vi "Test-Shoulder.vi"() -> ()   [LabVIEW 2023]
doc: "This VI implements the framework and scheduler for your robotics program. It should not be necessary to modify the framework. You are expected to add your code to the VIs called from Robot Main - the ones located in the Team Code folder within the project."
uses:
  <vilib>/Rock Robotics/WPI/DriverStation/WPI_DriverStationRobotMode2.ctl
  <vilib>/Rock Robotics/WPI/Simulation/Protocol/Devices/DriverStation/DS Update Ops.ctl
  <vilib>/Rock Robotics/WPI/ThirdParty/JAS_Junk/TrajLib/VI/DigSeqLogic_Edge_On.vi
  Robot Global Data.vi
  Shoulder/ShoulderCmdCalcSpeakerShootALWAYS.vi
  Shoulder/ShoulderCmdUpIncALWAYS.vi
  Shoulder/ShoulderCmdDownDecALWAYS.vi
  Shoulder/ShoulderCmdRestALWAYS.vi
  Shoulder/ShoulderCmdSpeakerShootALWAYS.vi
  Shoulder/ShoulderCmdStopALWAYS.vi
  Shoulder/ShoulderCmdAmpDeliverALWAYS.vi
panel:
  in  "CmdInc":bool
  in  "CmdDec":bool
  in  "CmdStop":bool
  out "Low Limit Switch":bool
  out "PosDeg":dbl format="%9.1f"
  in  "CmdRest":bool
  in  "CmdAmp":bool
  in  "CmdSpeaker":bool
  in  "CmdCalcSpeaker":bool
  out "Robot Mode":T1
  out "MotorOutDmd":dbl format="%9.2f"
  in  "error in (no error)":errorcluster
  in  "Finish":bool
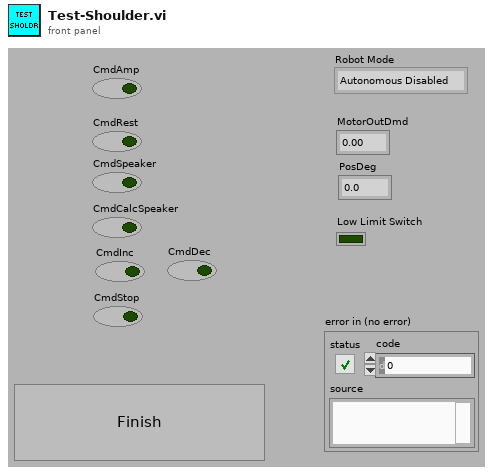
[diagram p1: front panel]
types:
  T1 = typedef "WPI_DriverStationRobotMode2.ctl" = enum16{"Autonomous Disabled", "Autonomous Enabled", "Teleop Disabled", "Teleop Enabled", "Disconnected", "Finish", "Test Disabled", "Test Enabled", "Emergency Stopped"}
  T2 = typedef "WPI_DriverStationMatch Info.ctl" = cluster{"Autonomous Elapsed Seconds":dbl, "TeleOp Elapsed Seconds":dbl, "Disabled Elapsed Seconds":dbl, "Visited Autonomous":bool, "Visited TeleOp":bool, "Visited Disabled":bool, "Autonomous Settings":cluster{"Autonomous Style":enum16{"Iterative", "Independent"}, "VI Refnum":refnum<vi>}}
  T3 = typedef "WPI_DriverStationDerivedRobotMode.ctl" = enum16{"Init", "Execute", "Stop"}
  T4 = typedef "DS Update Ops.ctl" = enum16{"set enabled", "set autonomous", "set test", "set estop", "set fms", "set ds", "set control word", "set match_time", "set station", "set game data", "JSON update", "set name", "get", "transmit initial", "reset"}
  T5 = typedef "NetComm_ControlWord.ctl" = cluster{"Enabled":bool, "Autonomous":bool, "Test":bool, "E-Stop":bool, "FMS Attached":bool, "DS Attached":bool}
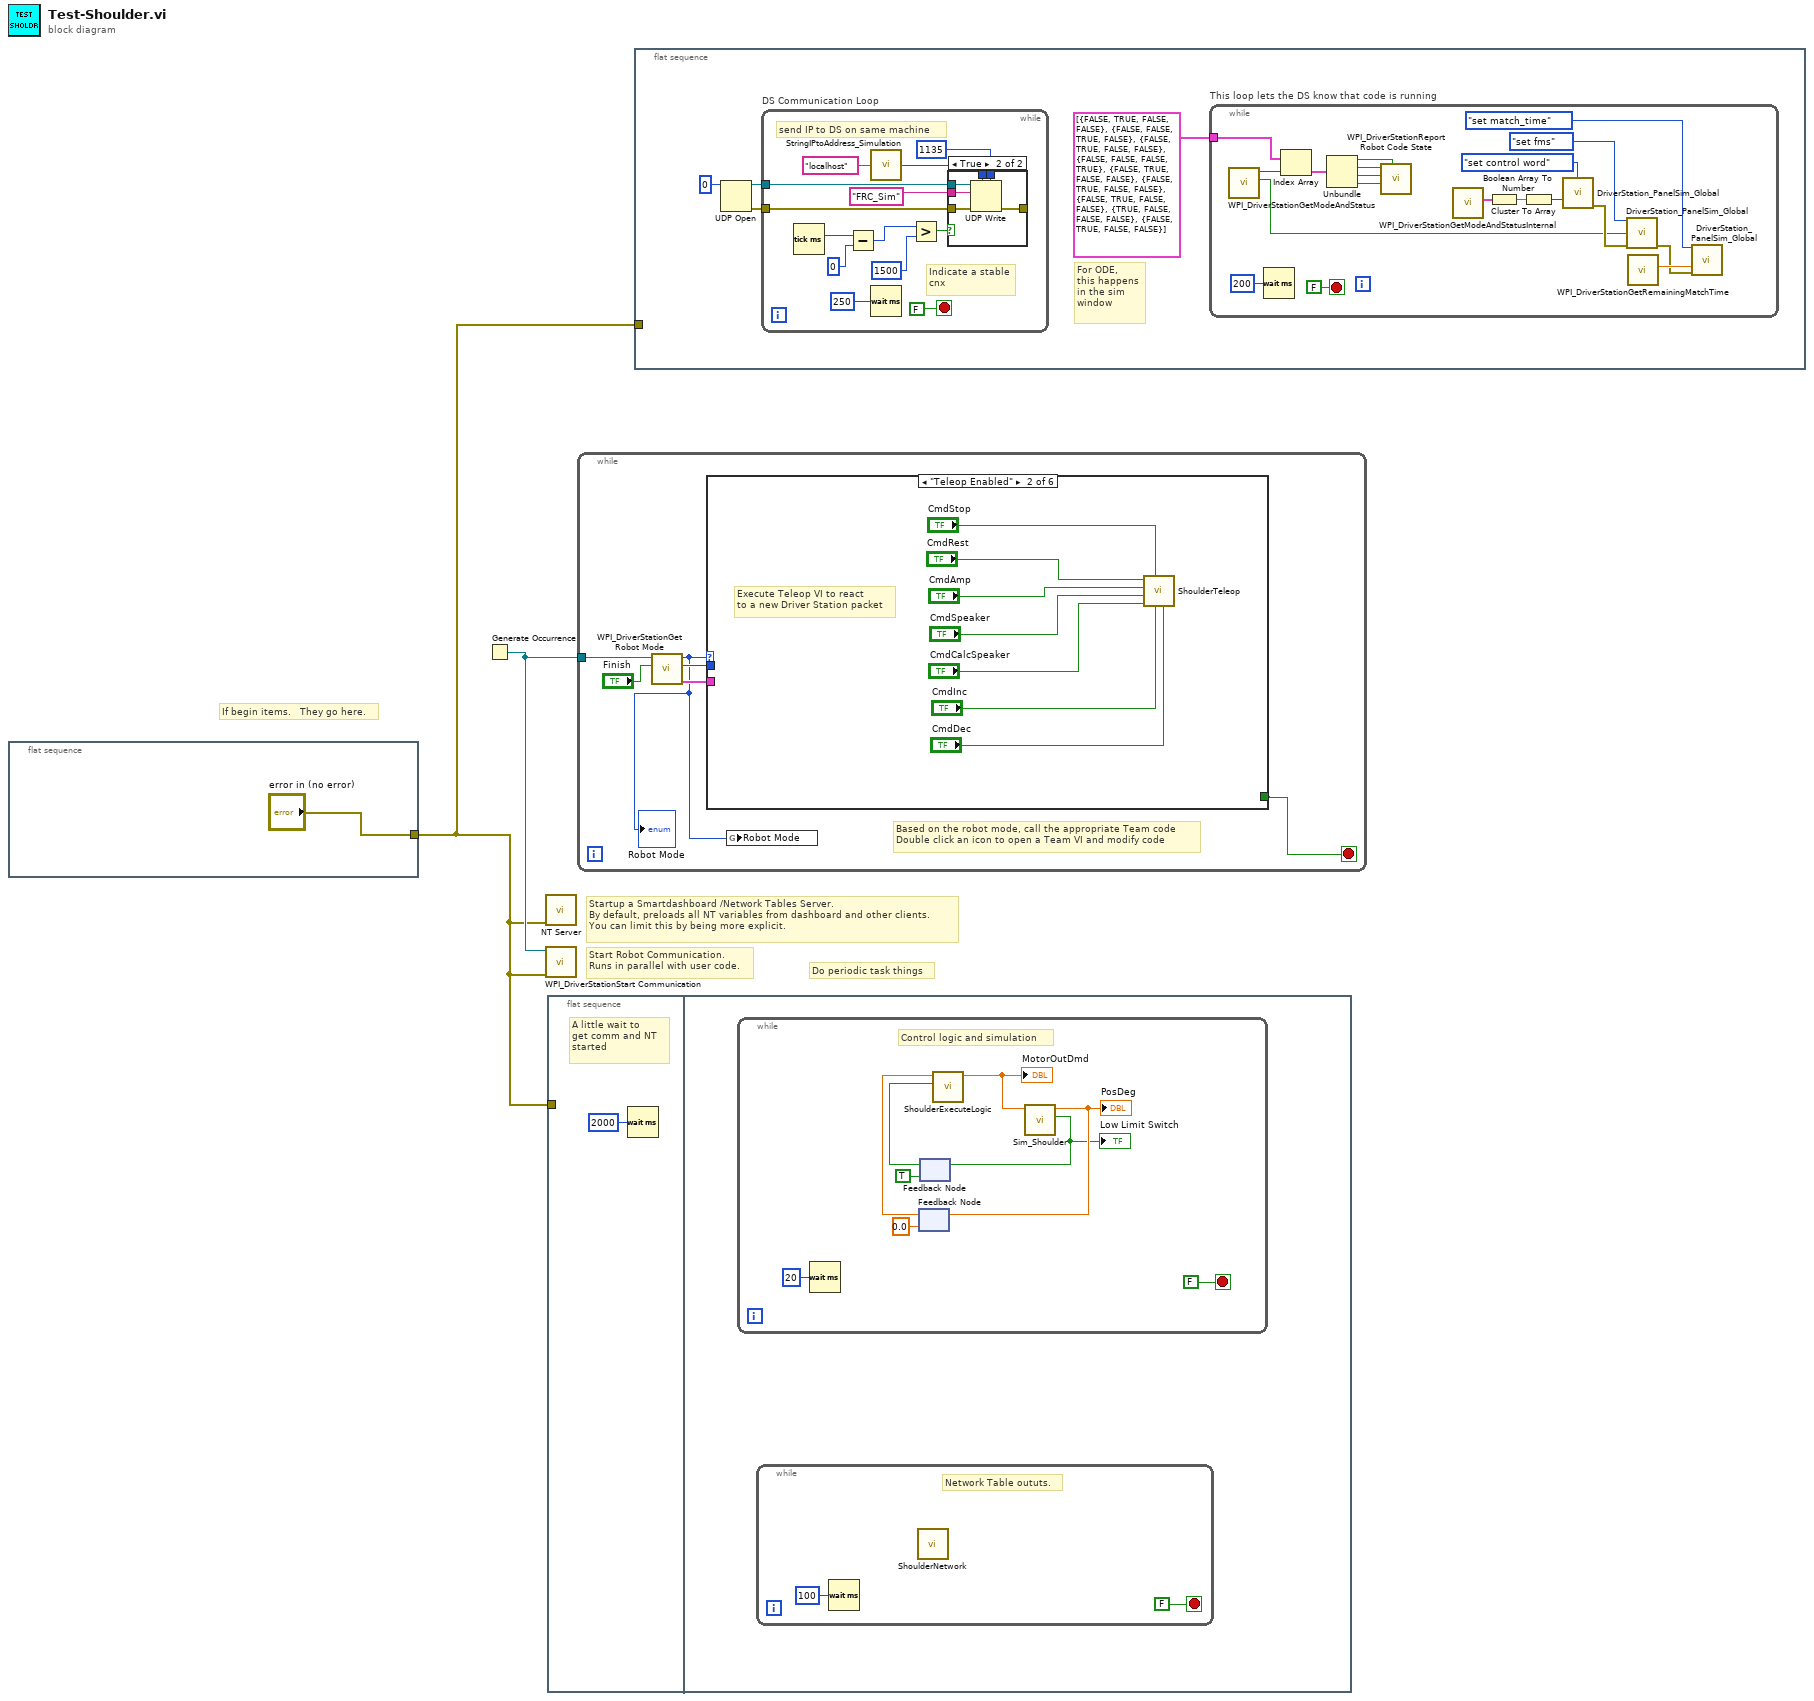
[diagram p0: block diagram]
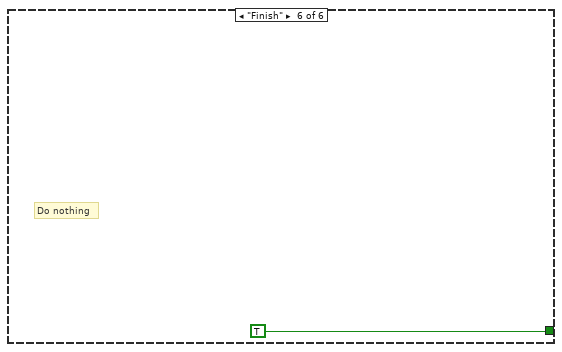
[diagram p6: hidden frame]
diagram:
  # "If begin items.   They go here."
  # "Do periodic task things"
  # "Startup a Smartdashboard /Network Tables Server.\nBy default, preloads all NT variables from dashboard and other clients.\nYou can limit this by being more explicit."
  # "Start Robot Communication.\nRuns in parallel with user code."
  n1 = flat-sequence {
    tunnel: ["error in (no error)"] -> w1
    frame #0 {
    }
  }
  n2 = Generate Occurrence() -> (w2:refnum<k4>)
  n3 = call <vilib>:"NT Server.vi"("error in (no error)"=w1) -> ()  [unwired: 10 in, 1 out]
  n4 = call <vilib>:"WPI_DriverStationStart Communication.vi"("error in (no error)"=w1, "occurrence"=w2) -> ()  [unwired: 1 in, 9 out]
  n5 = flat-sequence {
    tunnel: w1 -> [_]
    frame #0 {
      # "A little wait to\nget comm and NT\nstarted"
      n6 = Wait (ms)(milliseconds to wait=u32 2000) -> ()  [unwired: 1 out]
    }
    frame #1 {
      n7 = while {
        stop <- FALSE stop-if-true
        # "Control logic and simulation"
        n8 = Wait (ms)(milliseconds to wait=u32 20) -> ()  [unwired: 1 out]
        n9 = feedback #1(0.0 ("ArmPosDeg")) -> (w11:dbl)
        n10 = feedback #2(TRUE ("Low Limit Switch")) -> (w9:bool)
        n11 = call "ShoulderExecuteLogic.vi"("LowLimitSwitch"=w9, "PositionDeg"=w11) -> ("MotorDemand"=w13:dbl)  [unwired: 8 in, 1 out]
        "MotorOutDmd" <- w13
        n12 = call "Sim_Shoulder.vi"("Motor Dmd"=w13) -> ("Low Limit Switch"=w10:bool, "ArmPosDeg"=w12:dbl)  [unwired: 8 in, 1 out]
        "PosDeg" <- w12
        "Low Limit Switch" <- w10
        n13 = feedback-in #1(w12) -> ()
        n14 = feedback-in #2(w10) -> ()
      }
      n15 = while {
        stop <- FALSE stop-if-true
        # "Network Table oututs."
        n16 = Wait (ms)(milliseconds to wait=u32 100) -> ()  [unwired: 1 out]
        n17 = call "ShoulderNetwork.vi"() -> ()  [unwired: 11 in, 1 out]
      }
    }
  }
  n18 = while {
    tunnel: w2 -> [w21]
    stop <- w16 stop-if-true
    # "Based on the robot mode, call the appropriate Team code\nDouble click an icon to open a Team VI and modify code"
    n19 = call <vilib>:"WPI_DriverStationGet Robot Mode.vi"("Finish"="Finish", "DS Occurrence"=w21) -> ("Match Info out"=w18:T2, "Call Context"=w20:T3, "Robot Mode"=w17:T1)  [unwired: 7 out]
    "Robot Mode" <- w17
    n20 = case shown="\"Teleop Enabled\"" w17 {
      tunnel: w20 -> [_ _ _ _ _ _]
      tunnel: w18 -> [_ _ _ _ _ _]
      tunnel: [_ _ _ _ _ TRUE] -> w16
      frame "Autonomous Enabled" {
        # "Do nothing...."
      }
      frame "Teleop Enabled" {
        # "Execute Teleop VI to react\nto a new Driver Station packet"
        n21 = call "ShoulderTeleop.vi"("CmdDownDec"="CmdDec", "CmdUpInc"="CmdInc", "CmdStop"="CmdStop", "CmdCalcSpeaker"="CmdCalcSpeaker", "CmdSpeaker"="CmdSpeaker", "CmdAmp"="CmdAmp", "CmdRest"="CmdRest") -> ()  [unwired: 5 in]
      }
      frame "Test Disabled", "Test Enabled" {
        # "Do nothing"
      }
      frame "Autonomous Disabled", "Teleop Disabled" {
        # "Do nothing."
      }
      frame "Disconnected", Default {
        # "Driver Station packet didn't arrive.\nPossibly useful for diagnostics"
      }
      frame "Finish" {
        # "Do nothing"
      }
    }
    n22 = global write "Robot Global Data.vi" "Robot Mode"(w17) -> ()
  }
  n23 = flat-sequence {
    tunnel: w1 -> [_]
    frame #0 {
      # "For ODE,\nthis happens\nin the sim\nwindow"
      n24 = UDP Open(11:u16 0 ("port")) -> (port=w33:refnum<k16>, 0:w32:errorcluster)  [unwired: 4 in, 1 out]
      n25 = while "DS Communication Loop" {
        tunnel: w33 -> [w64]
        tunnel: w32 -> [w65]
        stop <- FALSE stop-if-true
        # "Indicate a stable\ncnx"
        # "send IP to DS on same machine"
        n26 = Tick Count (ms)() -> (millisecond timer value=w54:u32)
        n27 = Subtract(x=w54, y=u32 0) -> (x-y=w57:u32)
        n28 = call <vilib>:"StringIPtoAddress_Simulation.vi"("string IP"="localhost" ("DS IP 2")) -> ("address"=w61:u32)  [unwired: 14 in]
        n29 = Wait (ms)(milliseconds to wait=u32 250) -> ()  [unwired: 1 out]
        n30 = Greater?(x=w57, y=u32 1500 ("milliseconds to wait")) -> (0:w55:bool)
        n31 = case shown="True" w55 {
          tunnel: w65 -> [_ w71]
          tunnel: w64 -> [_ w70]
          tunnel: "FRC_Sim" ("data in") -> [_ w69]
          tunnel: w61 -> [_ w68]
          tunnel: [_ w67] -> _
          tunnel: u16 1135 ("port") -> [_ w66]
          frame False {
          }
          frame True {
            n32 = UDP Write(address=w68, port or service name=w66, connection ID=w70, data in=w69, 8:w71) -> (error out=w67:errorcluster)  [unwired: 1 in, 1 out]
          }
        }
      }
      n33 = while "This loop lets the DS know that code is running" {
        tunnel: cluster{bool, bool, bool, bool}[] [{FALSE, TRUE, FALSE, FALSE}, {FALSE, FALSE, TRUE, FALSE}, {FALSE, TRUE, FALSE, FALSE}, {FALSE, FALSE, FALSE, TRUE}, {FALSE, TRUE, FALSE, FALSE}, {FALSE, TRUE, FALSE, FALSE}, {FALSE, TRUE, FALSE, FALSE}, {TRUE, FALSE, FALSE, FALSE}, {FALSE, TRUE, FALSE, FALSE}] -> [w51]
        stop <- FALSE stop-if-true
        n34 = call <vilib>:"WPI_DriverStationGetModeAndStatus.vi"() -> ("FMS Attached"=w34:bool, "Robot Mode"=w45:T1)  [unwired: 10 in]
        n35 = Wait (ms)(milliseconds to wait=u32 200) -> ()  [unwired: 1 out]
        n36 = Index Array(array=w51, index=w45) -> (element=w46:cluster{bool, bool, bool, bool})
        n37 = Unbundle(w46) -> (w52:bool, w44:bool, w49:bool, w48:bool)
        n38 = call <vilib>:"WPI_DriverStationReport Robot Code State.vi"("Test"=w52, "TeleOp"=w48, "Autonomous"=w49, "Disabled"=w44) -> ()  [unwired: 7 in, 1 out]
        n39 = call <vilib>:"WPI_DriverStationGetModeAndStatusInternal.vi"() -> ("Control Word"=w42:T5)  [unwired: 10 in, 1 out]
        n40 = Cluster To Array(cluster=w42) -> (array=w41:bool[])
        n41 = Boolean Array To Number(Boolean array=w41) -> (number=w40:u32)
        n42 = call <vilib>:"DriverStation_PanelSim_Global.vi"("menu"=DS_Update_Ops."set control word", "Numeric Value"=w40) -> ("error out"=w38:errorcluster)  [unwired: 12 in, 1 out]
        n43 = call <vilib>:"DriverStation_PanelSim_Global.vi"("menu"=DS_Update_Ops."set fms", "Value Set"=w34, "error in (no error)"=w38) -> ("error out"=w35:errorcluster)  [unwired: 11 in, 1 out]
        n44 = call <vilib>:"WPI_DriverStationGetRemainingMatchTime.vi"() -> ("Match Time(s)"=w36:sgl)  [unwired: 10 in, 1 out]
        n45 = call <vilib>:"DriverStation_PanelSim_Global.vi"("menu"=DS_Update_Ops."set match_time", "Numeric Value"=w36, "error in (no error)"=w35) -> ()  [unwired: 11 in, 2 out]
      }
    }
  }
